vi "Read Configuration data0.vi"(8 "error in (no error)":errorcluster, 11 "Path":path) -> (0 "error out":errorcluster)   [LabVIEW 2020]
uses:
  <vilib>/Utility/config.llb/Read Key (Double).vi
  <vilib>/Utility/config.llb/Read Key (U32).vi
  <vilib>/Utility/config.llb/NI_LVConfig.lvlib
panel:
  out "Configuration Setting":T1={"offset"=0.0, "Signal Type"=enum."Sine Wave", "Amplitude"=1.0, "Frequency"=10.0, "Phase"=0.0, "Noise Amplitude "=1.0} {"Noise Amplitude" format="%.2p"; "Phase" format="%.2p"; "Frequency" format="%0.2p"; "Amplitude" format="%0.2p"; "offset" format="%0.2p"}
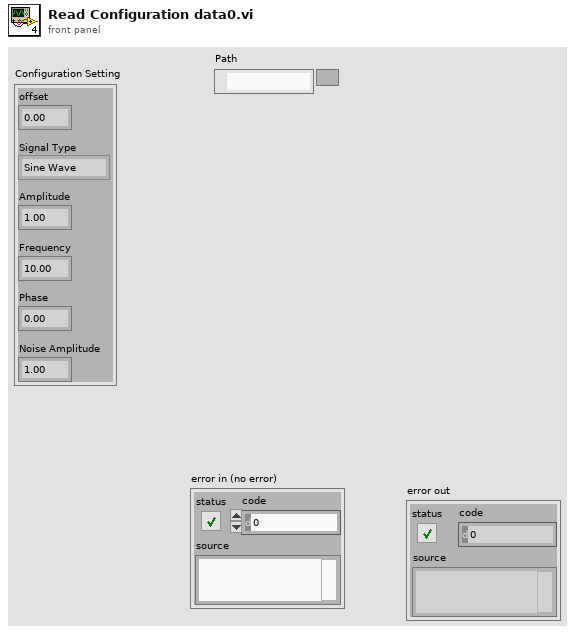
[diagram p1: front panel]
types:
  T1 = cluster{"offset":dbl, "Signal Type":enum16{"Sine Wave", "Triangle Wave", "Square Wave", "Sawtooth Wave"}, "Amplitude":dbl, "Frequency":dbl, "Phase":dbl, "Noise Amplitude ":dbl}
  T2 = enum16{"Sine Wave", "Triangle Wave", "Square Wave", "Sawtooth Wave"}
  T3 = typedef "NI_LVConfig.lvlib/Config Data RefNum.ctl" = refnum<k1>
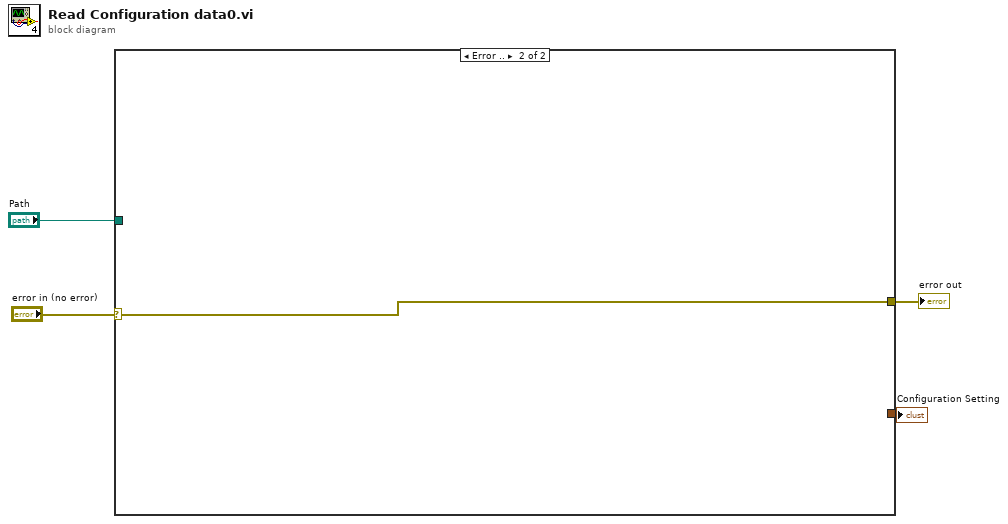
[diagram p0: block diagram]
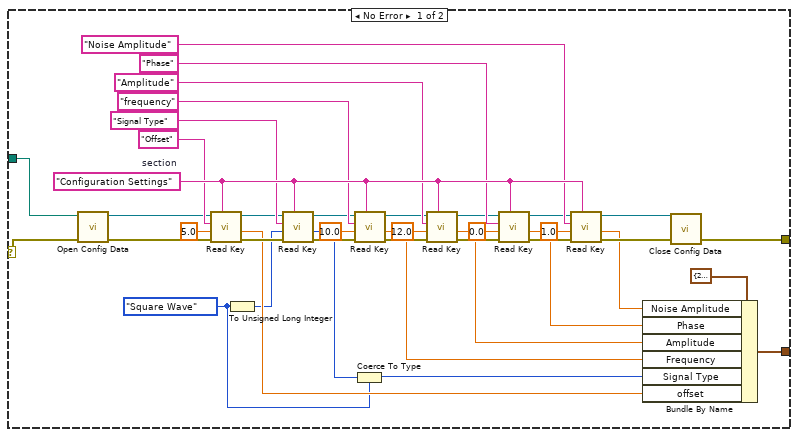
[diagram p2: hidden frame]
diagram:
  n1 = case shown="Error .." "error in (no error)" {
    selector: "error in (no error)" -> [w43 w45]
    tunnel: "Path" -> [w44 _]
    tunnel: [w42 w45] -> w2
    tunnel: [w40 _] -> w1
    frame No Error {
      w5 = T2."Square Wave" ("Signal Type")
      w39 = "Configuration Settings"  # section
      n2 = call <vilib>:"Open Config Data.vi"("error in (no error)"=w43, "configuration file path"=w44) -> ("error out"=w25:errorcluster, "refnum"=w26:T3)  [unwired: 7 in, 1 out]
      n3 = call-poly <vilib>:"Read Key.vi"("section"=w39, "error in (no error)"=w25, "default value"=5.0, "key"="Offset" ("section"), "refnum"=w26) -> ("error out"=w24:errorcluster, "value"=w18:dbl, "refnum out"=w32:T3)  [unwired: 3 in, 1 out]
      n4 = To Unsigned Long Integer(number=w5) -> (unsigned 32bit integer=w7:u32)
      n5 = call-poly <vilib>:"Read Key.vi"("section"=w39, "error in (no error)"=w24, "default value"=w7, "key"="Signal Type" ("section"), "refnum"=w32) -> ("error out"=w23:errorcluster, "value"=w17:u32, "refnum out"=w31:T3)  [unwired: 3 in, 1 out]
      n6 = Coerce To Type(0:w17, 1:w5) -> (2:w6:T2)
      n7 = call-poly <vilib>:"Read Key.vi"("section"=w39, "error in (no error)"=w23, "default value"=10.0, "key"="frequency" ("section"), "refnum"=w31) -> ("error out"=w22:errorcluster, "value"=w16:dbl, "refnum out"=w30:T3)  [unwired: 3 in, 1 out]
      n8 = call-poly <vilib>:"Read Key.vi"("section"=w39, "error in (no error)"=w22, "default value"=12.0, "key"="Amplitude" ("section"), "refnum"=w30) -> ("error out"=w21:errorcluster, "value"=w15:dbl, "refnum out"=w29:T3)  [unwired: 3 in, 1 out]
      n9 = call-poly <vilib>:"Read Key.vi"("section"=w39, "error in (no error)"=w21, "default value"=0.0, "key"="Phase" ("section"), "refnum"=w29) -> ("error out"=w20:errorcluster, "value"=w14:dbl, "refnum out"=w28:T3)  [unwired: 3 in, 1 out]
      n10 = call-poly <vilib>:"Read Key.vi"("section"=w39, "error in (no error)"=w20, "default value"=1.0, "key"="Noise Amplitude" ("section"), "refnum"=w28) -> ("error out"=w19:errorcluster, "value"=w13:dbl, "refnum out"=w27:T3)  [unwired: 3 in, 1 out]
      n11 = Bundle By Name(cluster=T1 {"offset"=2.0, "Signal Type"=enum."Sine Wave", "Amplitude"=10.0, "Frequency"=1000.0, "Phase"=50.0, "Noise Amplitude "=1.0} ("Configuration Setting"), "Noise Amplitude"=w13, "Phase"=w14, "Amplitude"=w15, "Frequency"=w16, "Signal Type"=w6, "offset"=w18) -> (w40:T1)
      n12 = call <vilib>:"Close Config Data.vi"("error in (no error)"=w19, "refnum"=w27) -> ("error out"=w42:errorcluster)  [unwired: 8 in, 1 out]
    }
    frame Error {
    }
  }
  "error out" <- w2
  "Configuration Setting" <- w1
